vi "EOL Printing_.vi"(6 "Print?":bool) -> ()   [LabVIEW 2018]
panel:
  out "error out":errorcluster
  in  "error in (no error)":errorcluster
  in  "DATA":string="E159914\n181120SD\n00001"
  in  "Path":path=path "D:/Valeo/Micriphone Test/UI/ME79.btw"
  in  "BarTender.IBtApplication":refnum<k7>
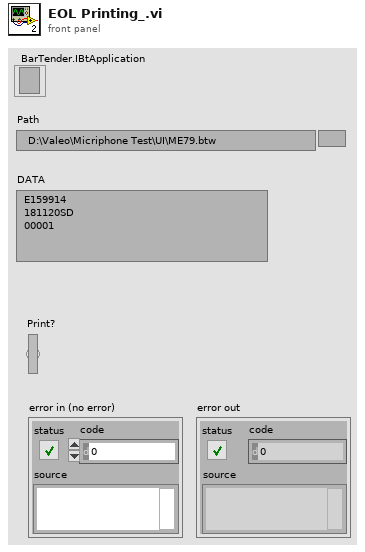
[diagram p1: front panel]
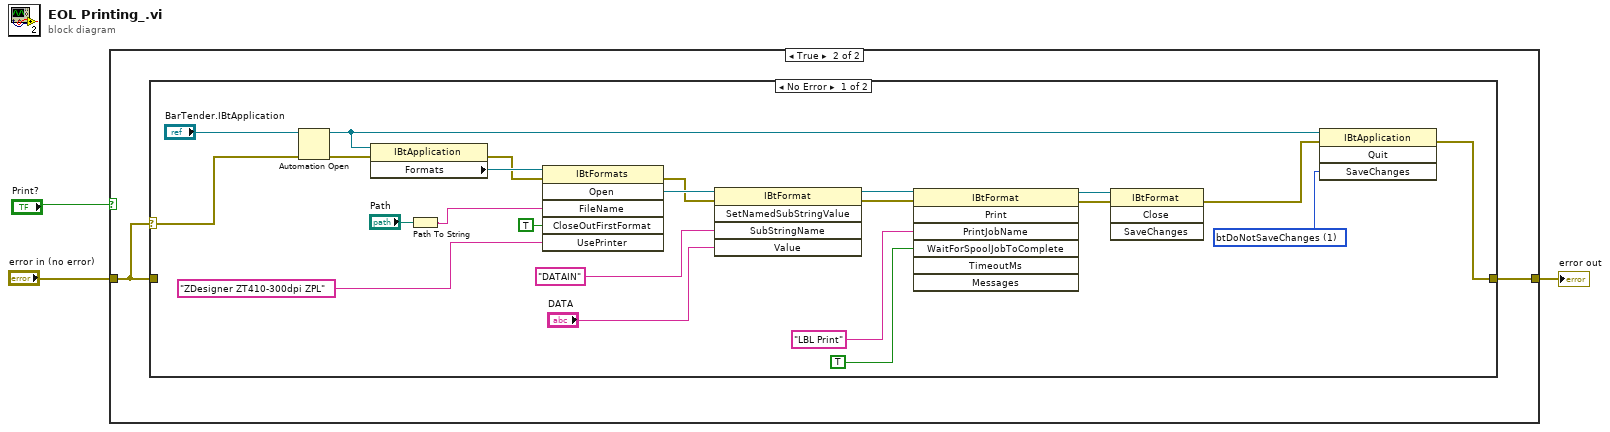
[diagram p0: block diagram]
diagram:
  n1 = case shown="True" "Print?" {
    tunnel: "error in (no error)" -> [w4 w5]
    tunnel: [w4 w6] -> w1
    frame False {
    }
    frame True {
      n2 = case shown="No Error" w5 {
        selector: w5 -> [w7 _]
        tunnel: [w8 w30] -> w6
        tunnel: w5 -> [_ w30]
        frame No Error {
          w21 = 1 items=["btPromptSave", "btDoNotSaveChanges", "btSaveChanges"] ("SaveChanges")
          n3 = Automation Open(error in (no error)=w7, Automation Refnum="BarTender.IBtApplication") -> (Automation Refnum=w22:refnum<k7>, error out=w28:errorcluster)  [unwired: 2 in]
          n4 = property class="IBtApplication"(reference=w22, error in=w28) -> (error out=w26:errorcluster, "Formats"=w27:refnum<k7>)  [unwired: 1 out]
          n5 = Path To String(path="Path") -> (string=w24:string)
          n6 = invoke class="IBtFormats" method="Open"(reference=w27, error in=w26, "FileName"=w24, "CloseOutFirstFormat"=TRUE, "UsePrinter"="ZDesigner ZT410-300dpi ZPL") -> (error out=w18:errorcluster, "Open"=w19:refnum<k7>)  [unwired: 1 in, 4 out]
          n7 = invoke class="IBtFormat" method="SetNamedSubStringValue"(reference=w19, error in=w18, "SubStringName"="DATAIN" ("FieldnameSampleDataList"), "Value"="DATA") -> (reference out=w16:refnum<k7>, error out=w17:errorcluster)  [unwired: 1 in, 3 out]
          n8 = invoke class="IBtFormat" method="Print"(reference=w16, error in=w17, "PrintJobName"="LBL Print", "WaitForSpoolJobToComplete"=TRUE) -> (reference out=w14:refnum<k7>, error out=w13:errorcluster)  [unwired: 3 in, 5 out]
          n9 = invoke class="IBtFormat" method="Close"(reference=w14, error in=w13) -> (error out=w12:errorcluster)  [unwired: 2 in, 3 out]
          n10 = invoke class="IBtApplication" method="Quit"(reference=w22, error in=w12, "SaveChanges"=w21) -> (error out=w8:errorcluster)  [unwired: 1 in, 3 out]
        }
        frame Error {
        }
      }
    }
  }
  "error out" <- w1
